vi "Read Accelerometers.vi"() -> (9 "myRIOAngle(x)":dbl, 11 "myRIOAngle(y)":dbl, 13 "myRIOAngle(z)":dbl, 14 "DrumAngle(x)":dbl, 15 "DrumAngle(y)":dbl, 16 "DrumAngle(z)":dbl, 17 "WinchAngle(x)":dbl, 18 "WinchAngle(y)":dbl, 19 "WinchAngle(z)":dbl)   [LabVIEW 2015]
uses:
  <vilib>/myRIO/Instrument Drivers/Onboard IO/I2C/typedefs/I2C User Configuration.ctl
  <vilib>/myRIO/Instrument Drivers/Onboard IO/I2C/typedefs/I2C Transfer Rate.ctl
  <vilib>/Platform/TimedLoop/XDataNode/timing_clust.ctl
  <vilib>/Platform/TimedLoop/XDataNode/nitl_modes.ctl
  <vilib>/Platform/TimedLoop/XDataNode/wakeup.ctl
  <vilib>/myRIO/Instrument Drivers/Onboard IO/I2C/typedefs/I2C Reference.ctl
  <vilib>/myRIO/Common/Instrument Driver Framework/Utilities/typedefs/myRIO Generic Hardware Reference.ctl
  <vilib>/myRIO/Common/Instrument Driver Framework/Utilities/typedefs/Hardware Version Enum.ctl
  <vilib>/myRIO/Common/Instrument Driver Framework/Utilities/typedefs/myRIO v1.0 Reference.ctl
  <vilib>/myRIO/Common/Instrument Driver Framework/Utilities/typedefs/Generic FPGA Reference.ctl
  <vilib>/myRIO/Common/Instrument Driver Framework/myRIO v1.0/I2C/typedefs/I2C Channels Enum.ctl
  <vilib>/myRIO/Instrument Drivers/Onboard IO/I2C/typedefs/I2C Configuration.ctl
  <vilib>/userdefined/High Color/nirio_resource_hc.ctl
  <vilib>/myRIO/Instrument Drivers/Onboard Devices/Accelerometer/typedefs/Accelerometer Reference.ctl
  <vilib>/myRIO/Common/Instrument Driver Framework/myRIO v1.0/Accelerometer/typedefs/Accelerometer Channels List.ctl
  <vilib>/myRIO/Common/Instrument Driver Framework/myRIO v1.0/Accelerometer/typedefs/Accelerometer Channels Enum.ctl
  <vilib>/myRIO/Common/Instrument Driver Framework/myRIO v1.0/I2C/vis/myRIO v1.1 Open I2C.vi
  <vilib>/myRIO/Common/Instrument Driver Framework/Utilities/vis/Is FPGA Ref Available.vi
  <vilib>/myRIO/Common/Instrument Driver Framework/myRIO v1.0/Accelerometer/vis/myRIO v1.1 Open Accelerometer.vi
  <vilib>/myRIO/Instrument Drivers/Onboard Devices/Accelerometer/vis/Read.vi
  <vilib>/myRIO/Common/Instrument Driver Framework/Utilities/vis/Validate Channels.vi
  <vilib>/myRIO/Common/Instrument Driver Framework/myRIO v1.0/I2C/vis/myRIO v1.0 Reserve I2C.vi
  <vilib>/myRIO/Common/Instrument Driver Framework/myRIO v1.0/Accelerometer/vis/myRIO v1.0 Reserve Accelerometer.vi
  <vilib>/myRIO/Common/Instrument Driver Framework/myRIO v1.0/I2C/vis/myRIO v1.0 Build MUX Configuration I2C.vi
  <vilib>/myRIO/Common/Instrument Driver Framework/myRIO v1.0/Resource Manager/vis/myRIO v1.0 Reserve Channel List.vi
  <vilib>/myRIO/Common/Instrument Driver Framework/myRIO v1.0/Accelerometer/vis/myRIO v1.0 Build MUX Configuration Accelerometer.vi
  <vilib>/myRIO/Common/Instrument Driver Framework/myRIO v1.0/Resource Manager/vis/myRIO v1.0 Create Configuration List.vi
  <vilib>/myRIO/Common/Instrument Driver Framework/myRIO v1.0/Resource Manager/vis/myRIO v1.0 Reserve Channel.vi
  <vilib>/myRIO/Common/Instrument Driver Framework/myRIO v1.0/Resource Manager/vis/myRIO v1.0 Unreserve Channel.vi
  <vilib>/myRIO/Common/Instrument Driver Framework/myRIO v1.0/Resource Manager/vis/myRIO v1.0 Build Mutex Name.vi
  <vilib>/Utility/VariantDataType/GetNumericInfo.vi
  <vilib>/Utility/error.llb/Error Cluster From Error Code.vi
  <vilib>/myRIO/Common/Instrument Driver Framework/myRIO v1.0/myRIO v1.1 Open.vi
  <vilib>/myRIO/Common/Instrument Driver Framework/Utilities/vis/IO Manager.vi
  <vilib>/myRIO/Common/Instrument Driver Framework/Utilities/vis/Configuration Manager.vi
  <vilib>/myRIO/Common/Instrument Driver Framework/myRIO v1.0/Resource Manager/vis/myRIO v1.0 Configure IO.vi
  <vilib>/myRIO/Common/Instrument Driver Framework/myRIO v1.0/myRIO v1.0 Close.vi
  <vilib>/myRIO/Common/Instrument Driver Framework/myRIO v1.0/I2C/vis/myRIO v1.0 Configure I2C.vi
  <vilib>/myRIO/Common/Instrument Driver Framework/myRIO v1.0/I2C/vis/myRIO v1.0 Write I2C.vi
  <vilib>/myRIO/Common/Instrument Driver Framework/myRIO v1.0/Accelerometer/vis/myRIO v1.0 Get Scaling Constant Accelerometer.vi
  <vilib>/myRIO/Common/Instrument Driver Framework/myRIO v1.0/Accelerometer/vis/myRIO v1.0 Read Accelerometer.vi
  <vilib>/myRIO/Common/Instrument Driver Framework/myRIO v1.0/I2C/vis/myRIO v1.0 Read I2C.vi
  <vilib>/Platform/TimedLoop/XDataNode/XDataNode.xnode
  <vilib>/myRIO/Instrument Drivers/Onboard IO/I2C/vis/myRIO I2C Open.xnode
  <vilib>/myRIO/Express VI/Onboard Devices/Accelerometer/Accelerometer Express VI.xnode
  <vilib>/myRIO/Instrument Drivers/Onboard Devices/Accelerometer/vis/myRIO Accelerometer Open.xnode
  <vilib>/myRIO/Instrument Drivers/Onboard IO/I2C/I2C.lvlib
  <vilib>/Platform/TimedLoop/XDataNode/XDNodeRunTimeDep.lvlib
  <vilib>/myRIO/Instrument Drivers/Onboard Devices/Accelerometer/Accelerometer.lvlib
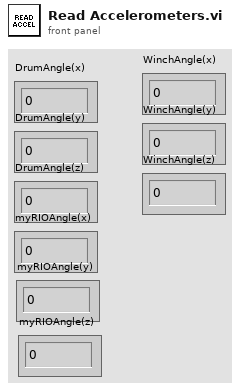
[diagram p1: front panel]
types:
  T1 = typedef "I2C.lvlib/I2C User Configuration.ctl" = cluster{"I2C Transfer Rate":T2}
  T2 = typedef "I2C.lvlib/I2C Transfer Rate.ctl" = enum16{"Standard mode (100 kbps)", "Fast mode (400 kbps)"}
  T3 = typedef "I2C.lvlib/I2C Reference.ctl" = cluster{"myRIO Reference":T4, "I2C Channels Enum":T8, "I2C Configuration":T9}
  T4 = typedef "myRIO Generic Hardware Reference.ctl" = cluster{"myRIO Model":T5, "myRIO Hardware Reference":T6}
  T5 = typedef "Hardware Version Enum.ctl" = enum16{"Unknown", "myRIO-1900", "myRIO-1950", "roboRIO"}
  T6 = typedef "myRIO v1.0 Reference.ctl" = cluster{"Generic FPGA Reference":T7, "Allow multiple opens":bool}
  T7 = typedef "Generic FPGA Reference.ctl" = refnum<k20>
  T8 = typedef "I2C Channels Enum.ctl" = enum16{"Not Connected", "A/I2C", "B/I2C", "I2C/I2C"}
  T9 = typedef "I2C.lvlib/I2C Configuration.ctl" = cluster{"I2C Transfer Rate":T2}
  T10 = typedef "XDNodeRunTimeDep.lvlib/timing_clust.ctl" = cluster{"Expected End [f-1]":u64, "Actual End [f-1]":u64, "Finished Late? [f-1]":bool, "Expected End [i-1]":u64, "Actual End [i-1]":u64, "Finished Late? [i-1]":bool, "Expected Start [i]":u64, "Actual Start [i]":u64, "Expected Start [f]":u64, "Actual Start [f]":u64, "Source Name":string, "Structure Name":string, "Period":i64, "Deadline":i64, "Offset":i64, "Start":i64, "Priority":i32, "Timeout":i32, "Mode":T11, "Wakeup Reason":T12, "Error":errorcluster, "Source Type":string, "Secondary Source Type":string, "Global End Time":u64, "Global Start Time":u64, "Frame Duration":u64, "Iteration Duration":u64, "Assigned CPU":i32, "I/O Scan Engine Mode":u32}
  T11 = typedef "XDNodeRunTimeDep.lvlib/nitl_modes.ctl" = enum32{"No Change", "Process missed periods, maintain original phase", "Discard missed periods, maintain original phase", "Process missed periods, ignore original phase", "Discard missed periods, ignore original phase"}
  T12 = typedef "XDNodeRunTimeDep.lvlib/wakeup.ctl" = enum32{"Normal", "Aborted", "Asynchronous wakeup", "Timing source error", "Timed loop error", "Timeout"}
  T13 = typedef "Accelerometer.lvlib/Accelerometer Reference.ctl" = cluster{"myRIO Reference":T4, "Accelerometer Channels List":T14, "LSB Weight":dbl}
  T14 = typedef "Accelerometer Channels List.ctl" = T15[]
  T15 = typedef "Accelerometer Channels Enum.ctl" = enum16{"Not Connected", "X-Axis", "Y-Axis", "Z-Axis"}
  T16 = typedef "nirio_resource_hc.ctl" = tag
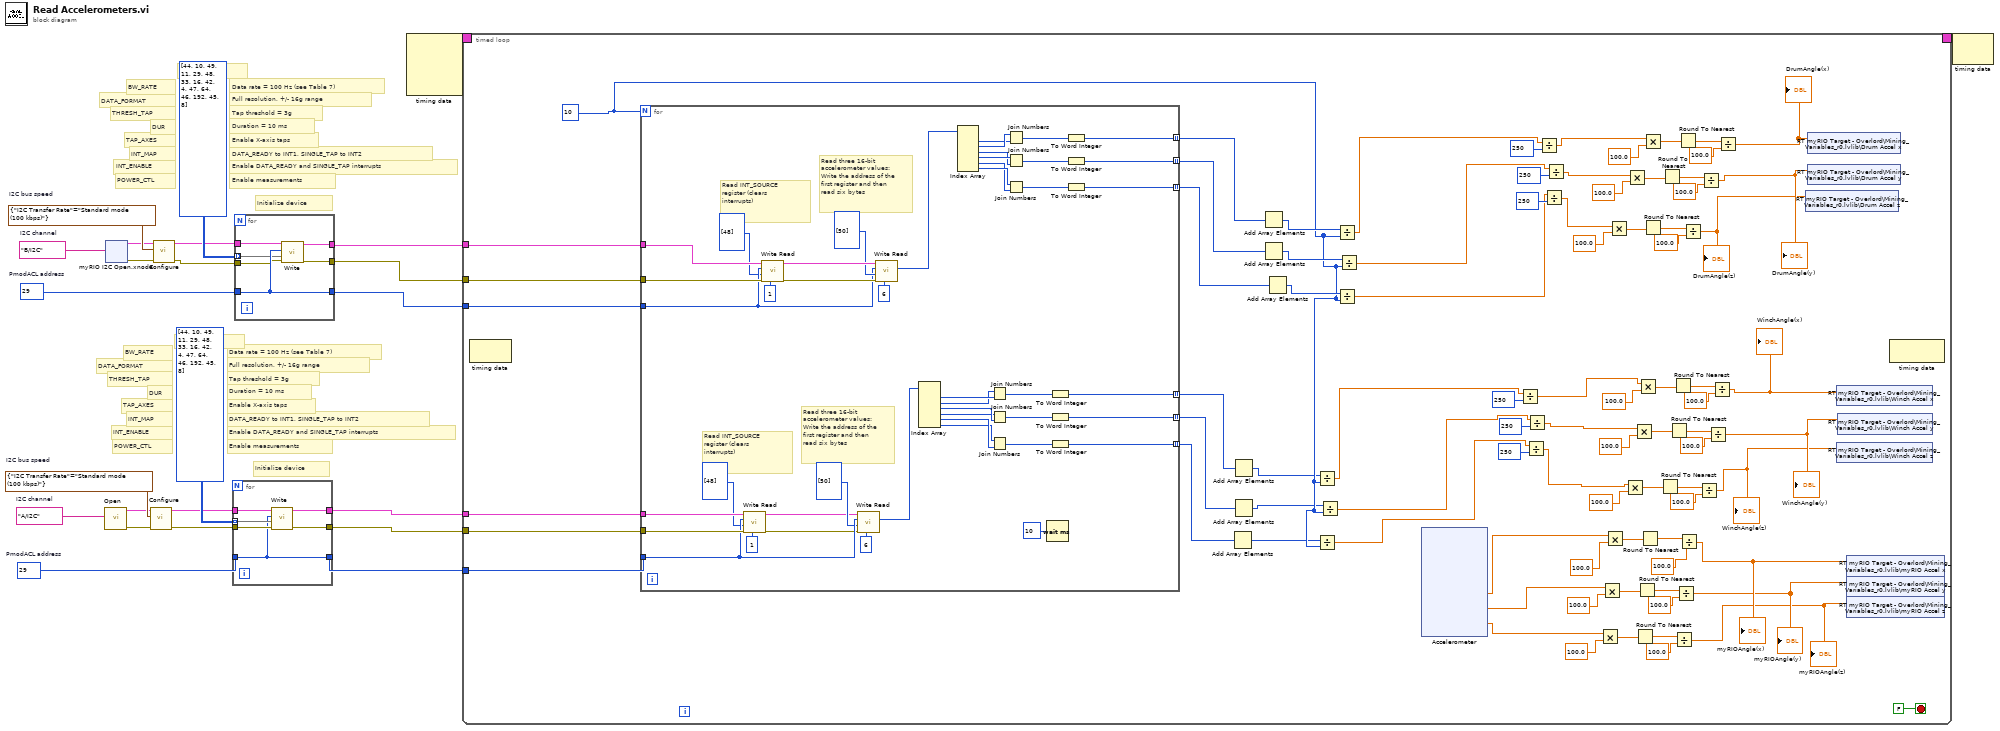
[diagram p0: block diagram]
diagram:
  w5 = T1 {"I2C Transfer Rate"=enum."Standard mode (100 kbps)"}  # I2C bus speed
  w6 = tag "B/I2C"  # I2C channel
  w10 = u8 29  # PmodACL address
  w23 = T1 {"I2C Transfer Rate"=enum."Standard mode (100 kbps)"}  # I2C bus speed
  w24 = tag "A/I2C"  # I2C channel
  w14 = u8 29  # PmodACL address
  # "Data rate = 100 Hz (see Table 7)"
  # "BW_RATE"
  # "DATA_READY to INT1, SINGLE_TAP to INT2"
  # "INT_MAP"
  # "Enable X-axis taps"
  # "TAP_AXES"
  # "Initialize device"
  # "Enable measurements"
  # "Enable DATA_READY and SINGLE_TAP interrupts"
  # "Duration = 10 ms"
  # "Tap threshold = 3g"
  # "POWER_CTL"
  # "INT_ENABLE"
  # "DUR"
  # "THRESH_TAP"
  # "Full resolution, +/- 16g range"
  # "DATA_FORMAT"
  # "register / data"
  # "Data rate = 100 Hz (see Table 7)"
  # "BW_RATE"
  # "DATA_READY to INT1, SINGLE_TAP to INT2"
  # "INT_MAP"
  # "Enable X-axis taps"
  # "TAP_AXES"
  # "Initialize device"
  # "Enable measurements"
  # "Enable DATA_READY and SINGLE_TAP interrupts"
  # "Duration = 10 ms"
  # "Tap threshold = 3g"
  # "POWER_CTL"
  # "INT_ENABLE"
  # "DUR"
  # "THRESH_TAP"
  # "Full resolution, +/- 16g range"
  # "DATA_FORMAT"
  # "register / data"
  n1 = call <vilib>:"Open.vi"("Channel Name"=w24) -> ("error out"=w21:errorcluster, "I2C Ref Out"=w22:T3)  [unwired: 9 in]
  n2 = xnode "myRIO I2C Open.xnode"("Channel Name"=w6) -> ("error out"=w3:errorcluster, "I2C Ref Out"=w4:T3)  [unwired: 2 in]
  n3 = call <vilib>:"Configure.vi"("error in (no error)"=w21, "I2C User Configuration"=w23, "I2C Ref In"=w22) -> ("error out"=w15:errorcluster, "I2C Ref Out"=w16:T3)  [unwired: 7 in]
  n4 = call <vilib>:"Configure.vi"("error in (no error)"=w3, "I2C User Configuration"=w5, "I2C Ref In"=w4) -> ("error out"=w1:errorcluster, "I2C Ref Out"=w2:T3)  [unwired: 7 in]
  n5 = for {
    tunnel: [w30] -> w20
    tunnel: [w29] -> w19
    tunnel: [w25] -> w18
    tunnel: u8[][] [[44, 10], [49, 11], [29, 48], [33, 16], [42, 4], [47, 64], [46, 192], [45, 8]] ("Bytes to Write") -> [w28] mode=indexing
    tunnel: w16 -> [w27]
    tunnel: w15 -> [w26]
    tunnel: w14 -> [w25]
    n6 = call <vilib>:"Write.vi"("error in (no error)"=w26, "Bytes to Write"=w28, "Slave Address (7-bit)"=w25, "I2C Ref In"=w27) -> ("error out"=w30:errorcluster, "I2C Ref Out"=w29:T3)  [unwired: 6 in]
  }
  n7 = for {
    tunnel: [w31] -> w8
    tunnel: [w32] -> w9
    tunnel: [w35] -> w7
    tunnel: u8[][] [[44, 10], [49, 11], [29, 48], [33, 16], [42, 4], [47, 64], [46, 192], [45, 8]] ("Bytes to Write") -> [w34] mode=indexing
    tunnel: w10 -> [w35]
    tunnel: w2 -> [w36]
    tunnel: w1 -> [w33]
    n8 = call <vilib>:"Write.vi"("error in (no error)"=w33, "Bytes to Write"=w34, "Slave Address (7-bit)"=w35, "I2C Ref In"=w36) -> ("error out"=w31:errorcluster, "I2C Ref Out"=w32:T3)  [unwired: 6 in]
  }
  n9 = node-c288() -> (w13:T10)  [unwired: 4 in]
  n10 = timed-loop "Timed Loop" {
    timing: w13 -> [_]
    timing-out: [_] -> w12
    tunnel: w20 -> [w122]
    tunnel: w19 -> [w121]
    tunnel: w18 -> [w120]
    tunnel: w9 -> [w112]
    tunnel: w8 -> [w111]
    tunnel: w7 -> [w110]
    stop <- FALSE stop-if-true
    w46 = 10
    n11 = node-c288() -> ()  [unwired: 1 in, 1 out]
    n12 = for {
      N: w46 -> [_]
      tunnel: w122 -> [w167]
      tunnel: w121 -> [w166]
      tunnel: w120 -> [w165]
      tunnel: [w148] -> w52 mode=indexing
      tunnel: [w147] -> w50 mode=indexing
      tunnel: [w146] -> w51 mode=indexing
      tunnel: [w145] -> w54 mode=indexing
      tunnel: [w144] -> w53 mode=indexing
      tunnel: [w143] -> w55 mode=indexing
      tunnel: w112 -> [w127]
      tunnel: w111 -> [w126]
      tunnel: w110 -> [w125]
      # "Read INT_SOURCE\nregister (clears\ninterrupts)"
      # "Read three 16-bit accelerometer values:\nWrite the address of the first register and then read six bytes"
      # "Read INT_SOURCE\nregister (clears\ninterrupts)"
      # "Read three 16-bit accelerometer values:\nWrite the address of the first register and then read six bytes"
      n13 = call <vilib>:"Write Read.vi"("Byte Count"=u32 1, "error in (no error)"=w167, "Bytes to Write"=u8[] [48], "Slave Address (7-bit)"=w165, "I2C Ref In"=w166) -> ("error out"=w150:errorcluster, "I2C Ref Out"=w151:T3)  [unwired: 3 in, 1 out]
      n14 = call <vilib>:"Write Read.vi"("Byte Count"=u32 1, "error in (no error)"=w126, "Bytes to Write"=u8[] [48], "Slave Address (7-bit)"=w125, "I2C Ref In"=w127) -> ("error out"=w141:errorcluster, "I2C Ref Out"=w140:T3)  [unwired: 3 in, 1 out]
      n15 = call <vilib>:"Write Read.vi"("Byte Count"=u32 6, "error in (no error)"=w150, "Bytes to Write"=u8[] [50], "Slave Address (7-bit)"=w165, "I2C Ref In"=w151) -> ("Bytes Read"=w149:u8[])  [unwired: 3 in, 2 out]
      n16 = call <vilib>:"Write Read.vi"("Byte Count"=u32 6, "error in (no error)"=w141, "Bytes to Write"=u8[] [50], "Slave Address (7-bit)"=w125, "I2C Ref In"=w140) -> ("Bytes Read"=w142:u8[])  [unwired: 3 in, 2 out]
      n17 = Index Array "Index Array"(array=w149) -> (element #1=w159:u8, element #2=w158:u8, element #3=w157:u8, element #4=w156:u8, element #5=w155:u8, element #6=w154:u8)  [unwired: 6 in]
      n18 = Index Array "Index Array"(array=w142) -> (element #1=w132:u8, element #2=w133:u8, element #3=w134:u8, element #4=w135:u8, element #5=w136:u8, element #6=w137:u8)  [unwired: 6 in]
      n19 = Join Numbers(hi=w158, lo=w159) -> ((hi.lo)=w164:u16)
      n20 = Join Numbers(hi=w156, lo=w157) -> ((hi.lo)=w163:u16)
      n21 = Join Numbers(hi=w154, lo=w155) -> ((hi.lo)=w162:u16)
      n22 = Join Numbers(hi=w133, lo=w132) -> ((hi.lo)=w128:u16)
      n23 = Join Numbers(hi=w135, lo=w134) -> ((hi.lo)=w129:u16)
      n24 = Join Numbers(hi=w137, lo=w136) -> ((hi.lo)=w130:u16)
      n25 = Wait (ms)(milliseconds to wait=u32 10) -> ()  [unwired: 1 out]
      n26 = To Word Integer(number=w164) -> (16bit integer=w148:i16)
      n27 = To Word Integer(number=w163) -> (16bit integer=w146:i16)
      n28 = To Word Integer(number=w162) -> (16bit integer=w147:i16)
      n29 = To Word Integer(number=w128) -> (16bit integer=w143:i16)
      n30 = To Word Integer(number=w129) -> (16bit integer=w145:i16)
      n31 = To Word Integer(number=w130) -> (16bit integer=w144:i16)
    }
    n32 = Add Array Elements(numeric array=w50) -> (sum=w43:i16)
    n33 = Add Array Elements(numeric array=w51) -> (sum=w44:i16)
    n34 = Add Array Elements(numeric array=w52) -> (sum=w45:i16)
    n35 = Add Array Elements(numeric array=w55) -> (sum=w49:i16)
    n36 = Add Array Elements(numeric array=w54) -> (sum=w48:i16)
    n37 = Add Array Elements(numeric array=w53) -> (sum=w47:i16)
    n38 = Divide(x=w45, y=w46) -> (x/y=w39:dbl)
    n39 = Divide(x=w43, y=w46) -> (x/y=w37:dbl)
    n40 = Divide(x=w44, y=w46) -> (x/y=w38:dbl)
    n41 = Divide(x=w49, y=w46) -> (x/y=w42:dbl)
    n42 = Divide(x=w47, y=w46) -> (x/y=w40:dbl)
    n43 = Divide(x=w48, y=w46) -> (x/y=w41:dbl)
    n44 = xnode "Accelerometer"() -> ("X-Axis"=w69:dbl, "Y-Axis"=w63:dbl, "Z-Axis"=w57:dbl)  [unwired: 1 in, 1 out]
    n45 = Divide(x=w39, y=i16 250) -> (x/y=w87:dbl)
    n46 = Divide(x=w37, y=i16 250) -> (x/y=w75:dbl)
    n47 = Divide(x=w38, y=i16 250) -> (x/y=w81:dbl)
    n48 = Divide(x=w42, y=i16 250) -> (x/y=w107:dbl)
    n49 = Divide(x=w40, y=i16 250) -> (x/y=w93:dbl)
    n50 = Divide(x=w41, y=i16 250) -> (x/y=w98:dbl)
    n51 = Multiply(x=w57, y=100.0) -> (x*y=w61:dbl)
    n52 = Multiply(x=w63, y=100.0) -> (x*y=w67:dbl)
    n53 = Multiply(x=w69, y=100.0) -> (x*y=w73:dbl)
    n54 = Multiply(x=w93, y=100.0) -> (x*y=w97:dbl)
    n55 = Multiply(x=w75, y=100.0) -> (x*y=w79:dbl)
    n56 = Multiply(x=w98, y=100.0) -> (x*y=w103:dbl)
    n57 = Multiply(x=w81, y=100.0) -> (x*y=w85:dbl)
    n58 = Round To Nearest(number=w61) -> (nearest integer value=w59:dbl)
    n59 = Round To Nearest(number=w67) -> (nearest integer value=w65:dbl)
    n60 = Multiply(x=w87, y=100.0) -> (x*y=w91:dbl)
    n61 = Round To Nearest(number=w73) -> (nearest integer value=w71:dbl)
    n62 = Multiply(x=w107, y=100.0) -> (x*y=w109:dbl)
    n63 = Round To Nearest(number=w97) -> (nearest integer value=w95:dbl)
    n64 = Round To Nearest(number=w79) -> (nearest integer value=w77:dbl)
    n65 = Round To Nearest(number=w103) -> (nearest integer value=w101:dbl)
    n66 = Round To Nearest(number=w85) -> (nearest integer value=w83:dbl)
    n67 = Round To Nearest(number=w91) -> (nearest integer value=w89:dbl)
    n68 = Divide(x=w59, y=100.0) -> (x/y=w56:dbl)
    "myRIOAngle(z)" <- w56
    n69 = Divide(x=w65, y=100.0) -> (x/y=w62:dbl)
    "myRIOAngle(y)" <- w62
    n70 = Round To Nearest(number=w109) -> (nearest integer value=w106:dbl)
    n71 = Divide(x=w71, y=100.0) -> (x/y=w68:dbl)
    "myRIOAngle(x)" <- w68
    n72 = Divide(x=w95, y=100.0) -> (x/y=w92:dbl)
    "DrumAngle(z)" <- w92
    n73 = Divide(x=w77, y=100.0) -> (x/y=w74:dbl)
    "WinchAngle(z)" <- w74
    n74 = Divide(x=w101, y=100.0) -> (x/y=w99:dbl)
    "DrumAngle(y)" <- w99
    n75 = Divide(x=w83, y=100.0) -> (x/y=w80:dbl)
    "WinchAngle(y)" <- w80
    n76 = Divide(x=w89, y=100.0) -> (x/y=w86:dbl)
    "WinchAngle(x)" <- w86
    n77 = Divide(x=w106, y=100.0) -> (x/y=w104:dbl)
    "DrumAngle(x)" <- w104
    n78 = shared-variable "RT myRIO Target - Overlord\\Mining_Variables_r0.lvlib\\Drum Accel z"(w92) -> ()  [unwired: 1 in, 1 out]
    n79 = shared-variable "RT myRIO Target - Overlord\\Mining_Variables_r0.lvlib\\Drum Accel x"(w104) -> ()  [unwired: 1 in, 1 out]
    n80 = shared-variable "RT myRIO Target - Overlord\\Mining_Variables_r0.lvlib\\Drum Accel y"(w99) -> ()  [unwired: 1 in, 1 out]
    n81 = shared-variable "RT myRIO Target - Overlord\\Mining_Variables_r0.lvlib\\Winch Accel x"(w86) -> ()  [unwired: 1 in, 1 out]
    n82 = shared-variable "RT myRIO Target - Overlord\\Mining_Variables_r0.lvlib\\Winch Accel z"(w74) -> ()  [unwired: 1 in, 1 out]
    n83 = shared-variable "RT myRIO Target - Overlord\\Mining_Variables_r0.lvlib\\Winch Accel y"(w80) -> ()  [unwired: 1 in, 1 out]
    n84 = shared-variable "RT myRIO Target - Overlord\\Mining_Variables_r0.lvlib\\myRIO Accel x"(w68) -> ()  [unwired: 1 in, 1 out]
    n85 = shared-variable "RT myRIO Target - Overlord\\Mining_Variables_r0.lvlib\\myRIO Accel y"(w62) -> ()  [unwired: 1 in, 1 out]
    n86 = shared-variable "RT myRIO Target - Overlord\\Mining_Variables_r0.lvlib\\myRIO Accel z"(w56) -> ()  [unwired: 1 in, 1 out]
    n87 = node-c288() -> ()  [unwired: 1 in, 1 out]
  }
  n88 = node-c288(w12) -> ()  [unwired: 1 out]
